vi "BindCtrlEvents.vi"(1 "Stop":refnum<vi>, 2 "VIs":refnum<vi>[](array[refnum]), 3 "Data":variant[](array[variant]), 4 "Type":T1=enum."Value Change", 5 "Ctrls":refnum<vi>[](array[refnum]), 6 "Names":string[](array[string])) -> (0 "Event":variant)   [LabVIEW 2014]
uses:
  <vilib>/event_ctls.llb/lveventtype.ctl
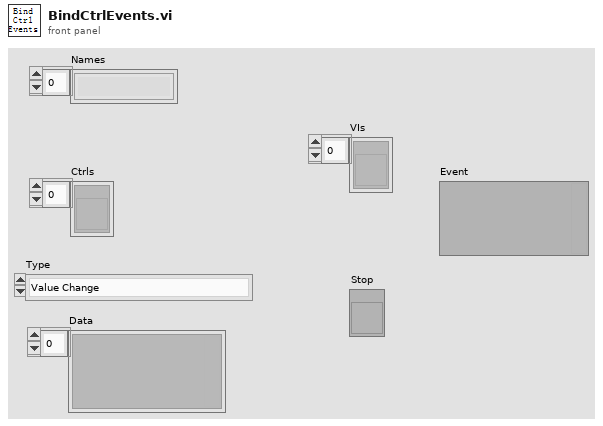
[diagram p1: front panel]
types:
  T1 = typedef "lveventtype.ctl" = enum32{"Null", "Timeout", "Annotation Menu Selection", "Annotation Menu Selection?", "App Instance Close", "App Instance Close?", "Autoscale Range Change", "Bookmark Info Change", "Cell Edit", "Cell Edit?", "Cursor Grab", "Cursor Grab?", "Cursor Menu Selection", "Cursor Menu Selection?", "Cursor Move", "Cursor Release", "Data Change", "Direction Change", "Display State Change", "Drag Ended", "Drag Enter", "Drag Leave", "Drag Over", "Drag Source Update", "Drag Starting", "Drag Starting?", "Drop", "Exec State Change", "Key Down", "Key Down?", "Key Repeat", "Key Repeat?", "Key Up", "Listbox Double Click", "Menu Activation?", "Menu Selection (App)", "Menu Selection? (App)", "Menu Selection (User)", "Mouse Down", "Mouse Down?", "Mouse Enter", "Mouse Leave", "Mouse Move", "Mouse Up", "Mouse Wheel", "NI Security User Change (App)", "Pane Size", "Panel Close", "Panel Close?", "Panel Resize", "Plot Attribute Change", "Scale Range Change", "Shortcut Menu Activation?", "Shortcut Menu Selection (App)", "Shortcut Menu Selection? (App)", "Shortcut Menu Selection (User)", "Tree Double Click", "Tree Drag", "Tree Drag?", "Tree Drop", "Tree Drop?", "Tree Item Close", "Tree Item Close?", "Tree Item Open", "Tree Item Open?", "User Event", "Value Change"}
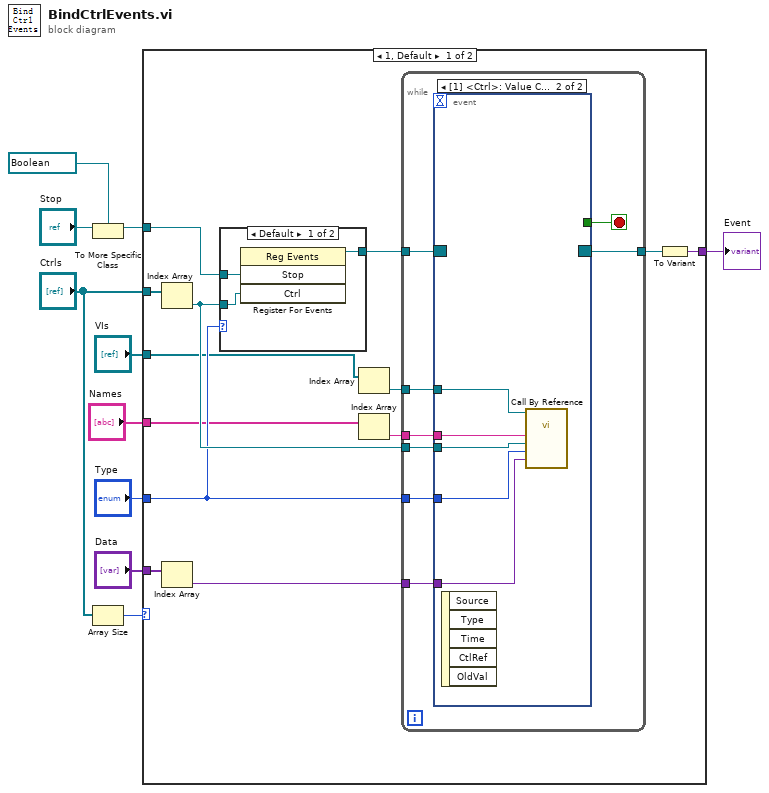
[diagram p0: block diagram]
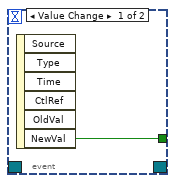
[diagram p2: hidden frame]
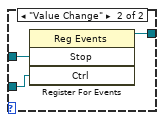
[diagram p3: hidden frame]
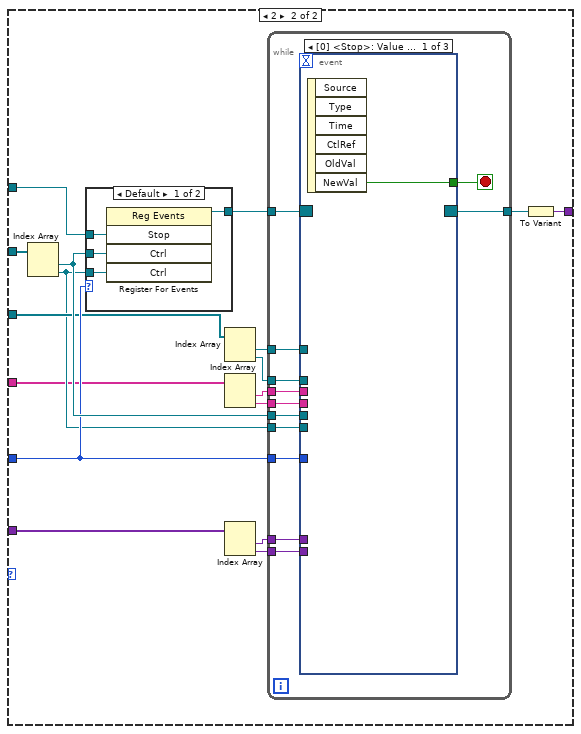
[diagram p4: hidden frame]
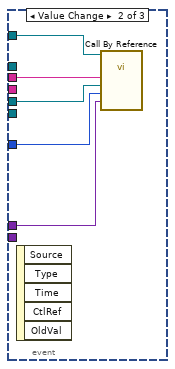
[diagram p5: hidden frame]
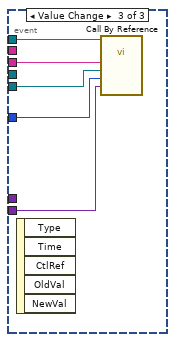
[diagram p6: hidden frame]
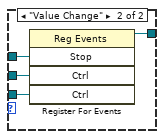
[diagram p7: hidden frame]
diagram:
  n1 = To More Specific Class(target class=refnum<vi> refnum ("Stop"), reference="Stop") -> (specific class reference=w2:refnum<vi>)  [unwired: 1 in, 1 out]
  n2 = Array Size(array="Ctrls") -> (size(s)=w10:i32)
  n3 = case shown="1, Default" w10 {
    tunnel: "Ctrls" -> [w23 w60]
    tunnel: "Type" -> [w21 w58]
    tunnel: "VIs" -> [w20 w57]
    tunnel: "Data" -> [w18 w55]
    tunnel: [w15 w49] -> w5
    tunnel: w2 -> [w14 w48]
    tunnel: "Names" -> [w12 w46]
    frame 1, Default {
      n4 = Index Array(array=w23) -> (element=w22:refnum<vi>)  [unwired: 1 in]
      n5 = Index Array(array=w18) -> (element=w17:variant)  [unwired: 1 in]
      n6 = case shown="Default" w21 {
        tunnel: w22 -> [w40 w43]
        tunnel: w14 -> [w39 w42]
        tunnel: [w38 w41] -> w13
        frame Default {
          n7 = register-events(w39, w40) -> (reference out=w38:refnum<event-registration>)  [unwired: 2 in, 1 out]
        }
        frame "Value Change" {
          n8 = register-events(w42, w43) -> (reference out=w41:refnum<event-registration>)  [unwired: 2 in, 1 out]
        }
      }
      n9 = Index Array(array=w20) -> (element=w19:refnum<vi>)  [unwired: 1 in]
      n10 = Index Array(array=w12) -> (element=w11:string)  [unwired: 1 in]
      n11 = while {
        tunnel: w22 -> [w31]
        tunnel: w21 -> [w30]
        tunnel: w19 -> [w29]
        tunnel: w17 -> [w28]
        tunnel: w13 -> [w26]
        tunnel: [w27] -> w16
        tunnel: w11 -> [w24]
        stop <- w25 stop-if-true
        n12 = event shown="[1] <Ctrl>: Value Change" {
          selector: w26 -> [_ _]
          dyn-events: [_ _] -> w27
          timeout: _ -> [_ _]
          tunnel: w31 -> [_ w35]
          tunnel: w30 -> [_ w34]
          tunnel: w28 -> [_ w33]
          tunnel: w29 -> [_ w37]
          tunnel: [w32 _] -> w25
          tunnel: w24 -> [_ w36]
          event Value Change {
            n13 = event-data() -> ("NewVal"=w32:bool)  [unwired: 1 in, 5 out]
          }
          event Value Change {
            n14 = event-data() -> ()  [unwired: 1 in, 5 out]
            n15 = call-by-ref "?"(reference=w37, "Data"=w33, "Type"=w34, "Ctrl"=w35, "Name"=w36) -> ()  [unwired: 1 in, 2 out]
          }
        }
      }
      n16 = To Variant(anything=w16) -> (Variant=w15:variant)
    }
    frame 2 {
      n17 = Index Array(array=w60) -> (element #1=w59:refnum<vi>, element #2=w52:refnum<vi>)  [unwired: 2 in]
      n18 = case shown="Default" w58 {
        tunnel: w59 -> [w86 w91]
        tunnel: w52 -> [w87 w90]
        tunnel: w48 -> [w85 w89]
        tunnel: [w84 w88] -> w47
        frame Default {
          n19 = register-events(w85, w86, w87) -> (reference out=w84:refnum<event-registration>)  [unwired: 2 in, 1 out]
        }
        frame "Value Change" {
          n20 = register-events(w89, w91, w90) -> (reference out=w88:refnum<event-registration>)  [unwired: 2 in, 1 out]
        }
      }
      n21 = Index Array(array=w57) -> (element #1=w56:refnum<vi>, element #2=w51:refnum<vi>)  [unwired: 2 in]
      n22 = Index Array(array=w46) -> (element #1=w44:string, element #2=w45:string)  [unwired: 2 in]
      n23 = Index Array(array=w55) -> (element #1=w54:variant, element #2=w53:variant)  [unwired: 2 in]
      n24 = while {
        tunnel: w59 -> [w72]
        tunnel: w58 -> [w71]
        tunnel: w56 -> [w70]
        tunnel: w54 -> [w69]
        tunnel: w53 -> [w68]
        tunnel: w52 -> [w67]
        tunnel: w51 -> [w66]
        tunnel: [w65] -> w50
        tunnel: w47 -> [w64]
        tunnel: w45 -> [w62]
        tunnel: w44 -> [w61]
        stop <- w63 stop-if-true
        n25 = event shown="[0] <Stop>: Value Change" {
          selector: w64 -> [_ _ _]
          dyn-events: [_ _ _] -> w65
          timeout: _ -> [_ _ _]
          tunnel: w72 -> [_ w76 _]
          tunnel: w71 -> [_ w75 w82]
          tunnel: w69 -> [_ w74 _]
          tunnel: w70 -> [_ w78 _]
          tunnel: w68 -> [_ _ w83]
          tunnel: w67 -> [_ _ w81]
          tunnel: w66 -> [_ _ w79]
          tunnel: [w73 _ _] -> w63
          tunnel: w62 -> [_ _ w80]
          tunnel: w61 -> [_ w77 _]
          event Value Change {
            n26 = event-data() -> ("NewVal"=w73:bool)  [unwired: 1 in, 5 out]
          }
          event Value Change {
            n27 = event-data() -> ()  [unwired: 1 in, 5 out]
            n28 = call-by-ref "?"(reference=w78, "Data"=w74, "Type"=w75, "Ctrl"=w76, "Name"=w77) -> ()  [unwired: 1 in, 2 out]
          }
          event Value Change {
            n29 = event-data() -> ()  [unwired: 1 in, 5 out]
            n30 = call-by-ref "?"(reference=w79, "Data"=w83, "Type"=w82, "Ctrl"=w81, "Name"=w80) -> ()  [unwired: 1 in, 2 out]
          }
        }
      }
      n31 = To Variant(anything=w50) -> (Variant=w49:variant)
    }
  }
  "Event" <- w5
